vi "Unroll states (SubVI).vi"(9 "size of each state":i32[](array[numeric]), 11 "State array":i32[](array[numeric])) -> (3 "Unrolled state":i32)   [LabVIEW 2013]
doc: "Unrolls a multi-dimension states to a 1D state. q = x + y*no.(x) + z*no.(x)*no.(y) + ... E.g. a given state (x, y, z) where x belongs to (0,99), y belongs to (0,59), z belongs to (0,1), then the state (2, 54, 23) it returns 143402."
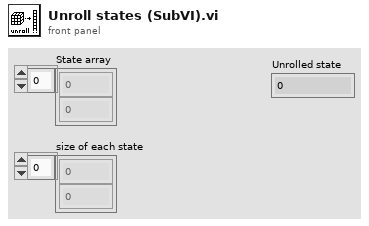
[diagram p1: front panel]
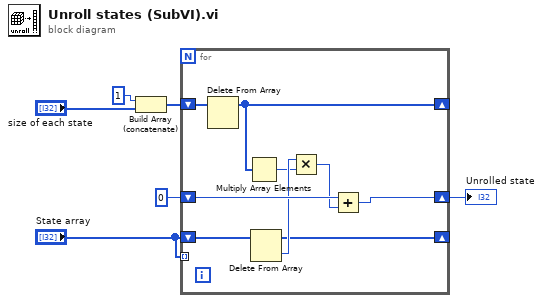
[diagram p0: block diagram]
diagram:
  n1 = Build Array (concatenate)(1, "size of each state") -> (w2:i32[])
  n2 = for {
    shift-right: [w8] -> _
    shift-left: w2 -> [w15]
    shift-right: [w13] -> w5
    shift-left: 0 -> [w12]
    tunnel: "State array" -> [_] mode=indexing
    shift-right: [w7] -> _
    shift-left: "State array" -> [w14]
    n3 = Delete From Array(array=w15) -> (array with subset deleted=w8:i32[])  [unwired: 2 in, 1 out]
    n4 = Multiply Array Elements(1:w8) -> (0:w9:i32)
    n5 = Delete From Array(array=w14) -> (deleted portion=w11:i32, array with subset deleted=w7:i32[])  [unwired: 2 in]
    n6 = Multiply(x=w11, y=w9) -> (x*y=w10:i32)
    n7 = Add(x=w12, y=w10) -> (x+y=w13:i32)
  }
  "Unrolled state" <- w5
